vi "Revision Query.vi"(0 "VISA resource name":refnum<visa-resource-name>, 5 "Unit Address (1)":u8=1, 11 "error in (no error)":errorcluster) -> (4 "VISA resource name out":refnum<visa-resource-name>, 8 "Instrument Driver Revision":string, 10 "Instrument Firmware Revision":string, 15 "error out":errorcluster)   [LabVIEW 2014, in "Eurotherm 35xx Series.lvlib"]
doc: "This VI queries the current instrument firmware revision and instrument driver revision.\n\nFor detailed driver information include modification history, refer to the et3500 Readme.html file."
uses:
  <instrlib>/Eurotherm 35xx Series/Eurotherm 35xx Series.lvlib
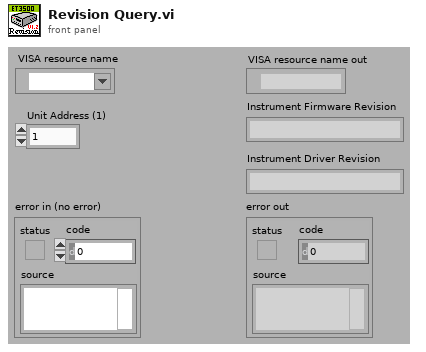
[diagram p1: front panel]
types:
  T1 = enum32{"invalid app kind", "Development System", "Run Time System", "Student Edition", "Embedded LabVIEW", "Evaluation", "Custom"}
  T2 = cluster{"Major":u16, "Minor":u16, "Fix":u16, "Build":u16}
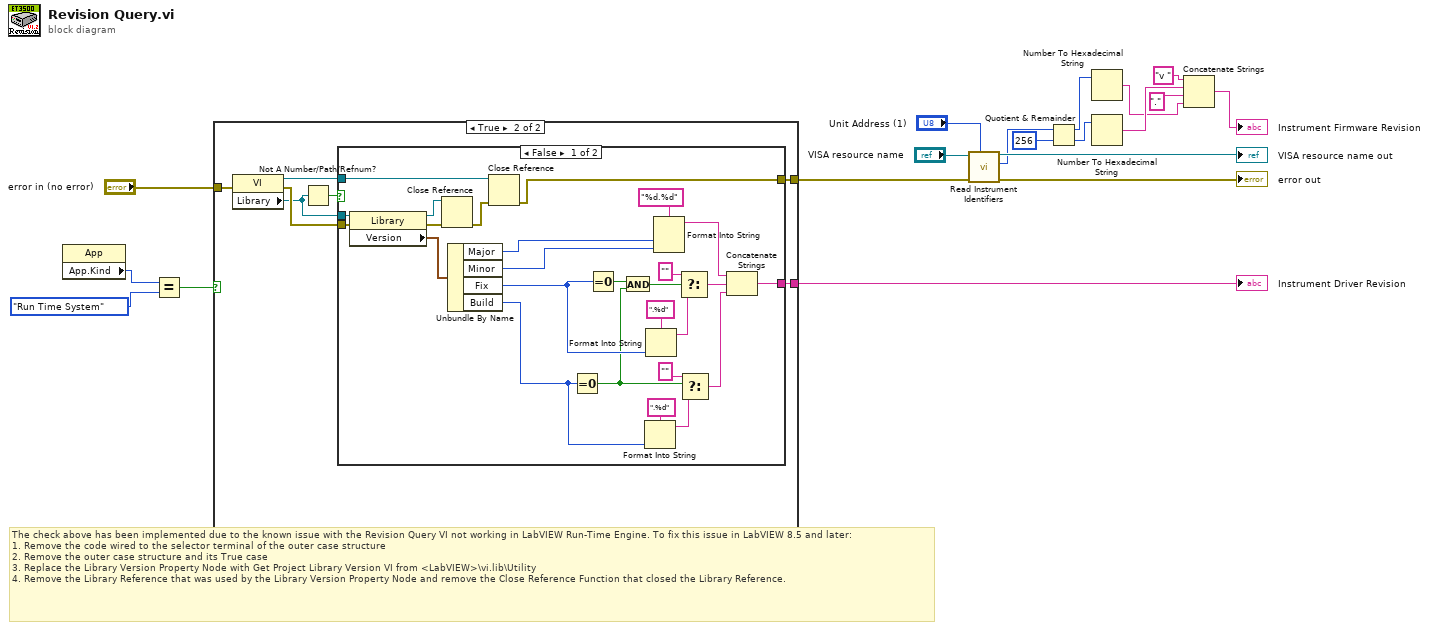
[diagram p0: block diagram]
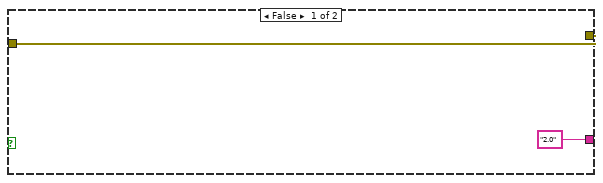
[diagram p2: hidden frame]
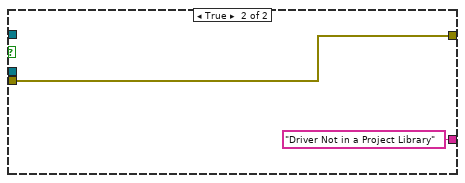
[diagram p3: hidden frame]
diagram:
  # "The check above has been implemented due to the known issue with the Revision Query VI not working in LabVIEW Run-Time Engine. To fix this issue in LabVIEW 8.5 and later:\n1. Remove the code wired to the selector terminal of the outer case structure\n2. Remove the outer case structure and its True case\n3. Replace the Library Version Property Node with Get Project Library Version VI from <LabVIEW>\\vi.lib\\Utility\n4. Remove the Library Reference that was used by the Library Version Property Node and remove the Close Reference Function that closed the Library Reference."
  n1 = property class="App"() -> ("App.Kind"=w3:T1)  [unwired: 2 in, 2 out]
  n2 = Equal?(x=w3, y=T1."Run Time System" ("Application:Kind")) -> (x = y?=w1:bool)
  n3 = case shown="True" w1 {
    tunnel: ["2.0" w24] -> w6
    tunnel: "error in (no error)" -> [w21 w23]
    tunnel: [w21 w22] -> w4
    frame False {
    }
    frame True {
      n4 = property class="VI"(error in=w23) -> (reference out=w28:refnum<vi>, error out=w27:errorcluster, "Library"=w26:refnum<vi>)  [unwired: 1 in]
      n5 = Not A Number/Path/Refnum?(number/path/refnum=w26) -> (NaN/Path/Refnum?=w25:bool)
      n6 = case shown="False" w25 {
        tunnel: w28 -> [w51 _]
        tunnel: w27 -> [w36 w56]
        tunnel: [w31 w56] -> w22
        tunnel: [w30 "Driver Not in a Project Library"] -> w24
        tunnel: w26 -> [w29 _]
        frame False {
          n7 = property class="Library"(reference=w29, error in=w36) -> (reference out=w53:refnum<vi>, error out=w54:errorcluster, "Version"=w50:T2)
          n8 = Close Reference(reference=w53, error in (no error)=w54) -> (error out=w52:errorcluster)
          n9 = Unbundle By Name(w50) -> ("Major"=w39:u16, "Minor"=w38:u16, "Fix"=w35:u16, "Build"=w37:u16)
          n10 = Close Reference(reference=w51, error in (no error)=w52) -> (error out=w31:errorcluster)
          n11 = Equal To 0?(x=w37) -> (x = 0?=w33:bool)
          n12 = Equal To 0?(x=w35) -> (x = 0?=w34:bool)
          n13 = And(x=w34, y=w33) -> (x .and. y?=w32:bool)
          n14 = Format Into String(format string=".%d", w37) -> (resulting string=w43:string)  [unwired: 2 in, 1 out]
          n15 = Format Into String(format string=".%d", w35) -> (resulting string=w47:string)  [unwired: 2 in, 1 out]
          n16 = Format Into String(format string="%d.%d", w39, w38) -> (resulting string=w45:string)  [unwired: 2 in, 1 out]
          n17 = Select(t="", s=w32, f=w47) -> (s? t:f=w44:string)
          n18 = Select(t="", s=w33, f=w43) -> (s? t:f=w40:string)
          n19 = Concatenate Strings(w45, w44, w40) -> (w30:string)
        }
        frame True {
        }
      }
    }
  }
  "Instrument Driver Revision" <- w6
  n20 = call <instrlib>:"Read Instrument Identifiers.vi"("Unit Address (1)"="Unit Address (1)", "error in (no error)"=w4, "VISA resource name"="VISA resource name") -> ("error out"=→"error out":errorcluster, "Instrument Version Number"=w13:u16, "VISA resource name out"=→"VISA resource name out":refnum<visa-resource-name>)  [unwired: 3 in, 3 out]
  n21 = Quotient & Remainder(x=w13, y=u16 256) -> (x-y*floor(x/y)=w11:u16, floor(x/y)=w10:u16)
  n22 = Number To Hexadecimal String(2:w11) -> (0:w8:string)  [unwired: 1 in]
  n23 = Number To Hexadecimal String(2:w10) -> (0:w9:string)  [unwired: 1 in]
  n24 = Concatenate Strings("v " ("string"), w9, "." ("Instrument Firmware Revision"), w8) -> (→"Instrument Firmware Revision":string)
